vi "UpdateUI.vi"(8 "Error In":errorcluster, 10 "FeedbackData":T1, 11 "ManualModeUIRefs":T2) -> (0 "Error Out":errorcluster)   [LabVIEW 2019, in "ManualMode.lvlib"]
uses:
  ManualMode.lvlib
  Cluster - UIRefs.ctl
  Mark10 API/Cluster - FeedbackData.ctl
  Mark10 API/Mark 10 TSTM-DC.lvlib
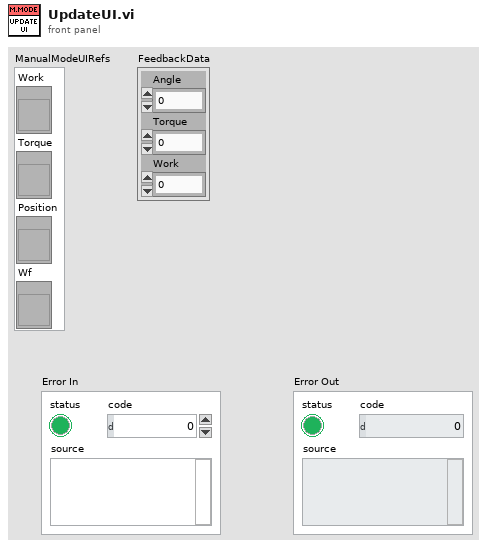
[diagram p1: front panel]
types:
  T1 = typedef "Mark 10 TSTM-DC.lvlib/Cluster - FeedbackData.ctl" = cluster{"Angle":dbl, "Torque":dbl, "Work":dbl}
  T2 = typedef "ManualMode.lvlib/Cluster - UIRefs.ctl" = cluster{"Work":refnum<vi>, "Torque":refnum<vi>, "Position":refnum<vi>, "Wf":refnum<vi>}
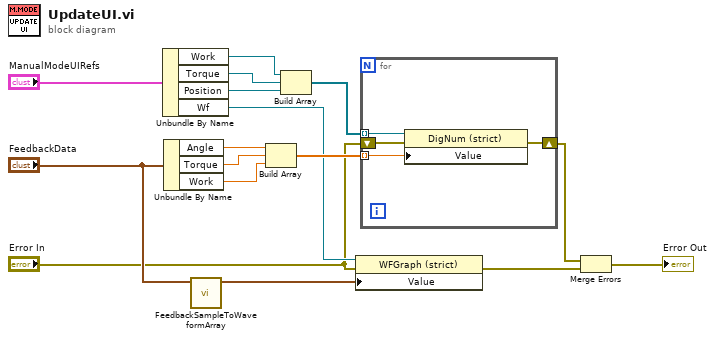
[diagram p0: block diagram]
diagram:
  n1 = Unbundle By Name("ManualModeUIRefs") -> ("Work"=w9:refnum<vi>, "Torque"=w10:refnum<vi>, "Position"=w15:refnum<vi>, "Wf"=w6:refnum<vi>)
  n2 = Unbundle By Name("FeedbackData") -> ("Angle"=w14:dbl, "Torque"=w13:dbl, "Work"=w12:dbl)
  n3 = call "FeedbackSampleToWaveformArray.vi"("FeedbackData"="FeedbackData") -> ("WfArray"=w5:waveform(dbl)[])  [unwired: 10 in]
  n4 = Build Array(w14, w13, w12) -> (w8:dbl[])
  n5 = Build Array(w9, w10, w15) -> (w11:refnum<vi>[])
  n6 = property class="WFGraph (strict)"(reference=w6, error in="Error In", "Value"=w5) -> (error out=w2:errorcluster)  [unwired: 1 out]
  n7 = for {
    tunnel: w11 -> [w20] mode=indexing
    tunnel: w8 -> [w19] mode=indexing
    shift-right: [w17] -> w3
    shift-left: "Error In" -> [w18]
    n8 = property class="DigNum (strict)"(reference=w20, error in=w18, "Value"=w19) -> (error out=w17:errorcluster)  [unwired: 1 out]
  }
  n9 = Merge Errors(w3, w2) -> (→"Error Out":errorcluster)
